vi "Write Log Filter.vi"(8 "error in (no error)":errorcluster, 10 "Log Filter":refnum<class "ILogFilter.lvclass">, 11 "Log Sink in":refnum<class "Log Sink.lvclass">) -> (0 "error out":errorcluster, 3 "Log Sink out":refnum<class "Log Sink.lvclass">)   [LabVIEW 2020, in "Composed Log.lvlib" / "Log Sink.lvclass"]
uses:
  <vilib>/gpm_packages/@cs/event-logger/Source/Composed Log/Log Sink/Log Sink.lvclass
  <vilib>/gpm_packages/@cs/event-logger/Source/Composed Log/ILogFilter/ILogFilter.lvclass
  <vilib>/gpm_packages/@cs/event-logger/Source/Composed Log/Log Sink/Log Sink.lvclass/Log Sink.ctl
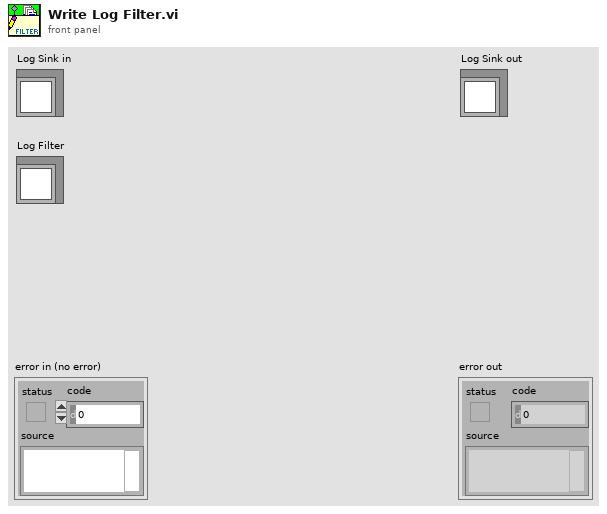
[diagram p1: front panel]
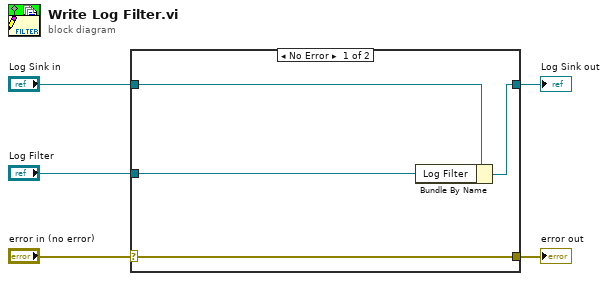
[diagram p0: block diagram]
diagram:
  n1 = case shown="No Error" "error in (no error)" {
    selector: "error in (no error)" -> [w9 w10]
    tunnel: [w9 w10] -> w4
    tunnel: [w7 w11] -> w2
    tunnel: "Log Sink in" -> [w8 w11]
    tunnel: "Log Filter" -> [w6 _]
    frame No Error {
      n2 = Bundle By Name(cluster=w8, "Log Filter"=w6) -> (w7:refnum<class "Log Sink.lvclass">)
    }
    frame Error {
    }
  }
  "error out" <- w4
  "Log Sink out" <- w2
